vi "test Loopback BC to RT with Start and Stop.vi"(8 "error in":errorcluster, 11 "TestCase in":refnum<class "Loopback.lvclass">) -> (0 "error out":errorcluster, 3 "TestCase out":refnum<class "Loopback.lvclass">)   [LabVIEW 2020, in "Loopback.lvclass"]
uses:
  Loopback.lvclass
  C:/Git/niveristand-custom-device-testing-tools/VeriStandTestCase/VeriStandTestCase.lvclass
  <vilib>/numeric/Random Number (Range) U64.vi
  485b7c2b-8320-4722-9ec7-d01f27c65546.vi
  b08989c6-5f8b-4abd-9880-ddf65696a96d.vi
  632f36f1-4b6f-4095-917c-563c19b80c3a.vi
  c8f491d9-e213-4f8e-8b18-a73afe23b1be.vi
  0f9dda61-2c21-4955-8588-a8fc95227647.vi
  33c3b3d1-f053-43c7-bbe8-20c4ad88f1fe.vi
  757b3fb2-d48b-4fbb-8961-a38cd8e327a9.vi
  ff2cfcab-6673-4a18-a151-e28207f633c9.vi
  9a38d044-f7fa-4f05-ac83-bb7c785194b9.vi
  <vilib>/numeric/sub_Random U32.vi
  <vilib>/NI VeriStand/Execution/Workspace/NI VeriStand - Set Multiple Channel Values.vi
  <vilib>/NI VeriStand/Execution/Workspace/NI VeriStand - Get Multiple Channel Values.vi
  <vilib>/NI VeriStand/Execution/Workspace/NI VeriStand - Set Single Channel Value.vi
  <vilib>/addons/_JKI Toolkits/VI Tester/TestCase.llb/TestCase.lvclass
  <vilib>/NI VeriStand/Execution/Workspace/NI_VS Workspace ExecutionAPI.lvlib
  C:/Program Files (x86)/National Instruments/LabVIEW 2020/vi.lib/addons/_JKI Toolkits/VI Tester/TestCase.llb/TestCase.lvclass
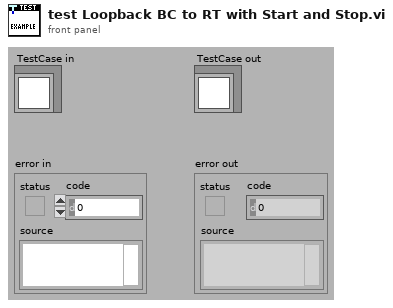
[diagram p1: front panel]
types:
  T1 = typedef "NI_VS Workspace ExecutionAPI.lvlib/WorkspaceAPI.ctl" = refnum<k24>
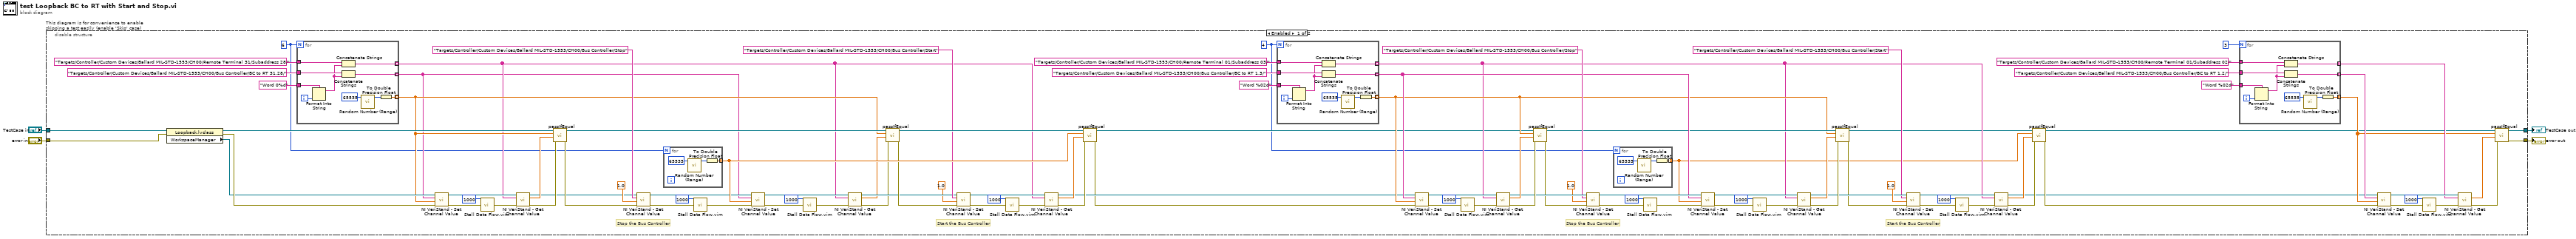
[diagram p0: block diagram]
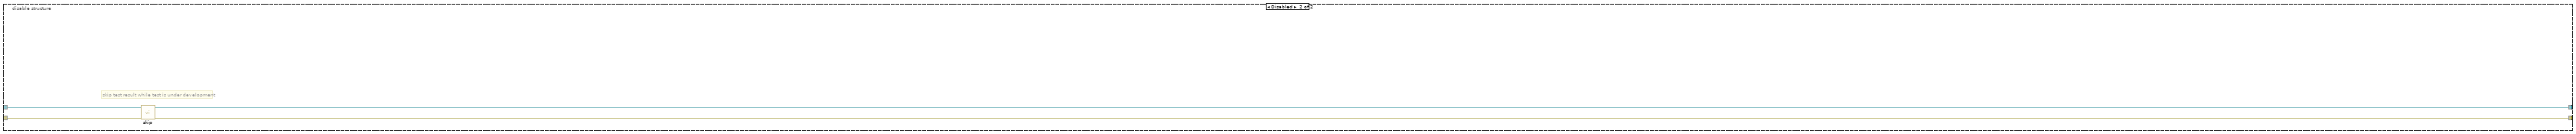
[diagram p2: hidden frame]
diagram:
  n1 = disable-structure "This diagram is for convenience to enable skipping a test easily (enable 'Skip' case)" shown="Enabled" {
    disable-tunnel: "TestCase in" -> [w101 w150]
    disable-tunnel: [w74 w148] -> w1
    disable-tunnel: [w73 w149] -> w3
    disable-tunnel: "error in" -> [w98 w147]
    frame Enabled {
      w5 = 4
      w6 = 6
      # "Start the Bus Controller"
      # "Stop the Bus Controller"
      # "Start the Bus Controller"
      # "Stop the Bus Controller"
      n2 = property class="Loopback.lvclass"(reference=w101, error in=w98) -> (reference out=w110:refnum<class "Loopback.lvclass">, error out=w105:errorcluster, "WorkspaceManager"=w103:T1)
      n3 = for {
        N: w6 -> [_]
        tunnel: "Targets/Controller/Custom Devices/Ballard MIL-STD-1553/CH00/Bus Controller/BC to RT 31.28/" ("Channel") -> [w145]
        tunnel: [w146] -> w8 mode=indexing
        tunnel: "Targets/Controller/Custom Devices/Ballard MIL-STD-1553/CH00/Remote Terminal 31/Subaddress 28/" ("Channel") -> [w144]
        tunnel: [w143] -> w9 mode=indexing
        tunnel: "Word 0%d" -> [w141]
        tunnel: [w137] -> w10 mode=indexing
        i -> [w142]
        n4 = Format Into String(format string=w141, w142) -> (resulting string=w140:string)  [unwired: 2 in, 1 out]
        n5 = Concatenate Strings(w144, w140) -> (w143:string)
        n6 = Concatenate Strings(w145, w140) -> (w146:string)
        n7 = call-poly <vilib>:"Random Number (Range).vi"("upper bound (100)"=u64 65535) -> ("number"=w139:u64)  [unwired: 10 in]
        n8 = To Double Precision Float(number=w139) -> (double precision float=w137:dbl)
      }
      n9 = call-poly <vilib>:"NI VeriStand - Set Channel Value.vi"("error in (no error)"=w105, "Values"=w10, "Channels"=w8, "WorkspaceManager in"=w103) -> ("error out"=w107:errorcluster, "WorkspaceManager out"=w109:T1)  [unwired: 6 in]
      n10 = call "Stall Data Flow.vim"("value in"=w107, "milliseconds to wait"=u32 1000) -> ("value out"=w108:errorcluster)  [unwired: 1 out]
      n11 = call-poly <vilib>:"NI VeriStand - Get Channel Value.vi"("error in (no error)"=w108, "Channels"=w9, "WorkspaceManager in"=w109) -> ("error out"=w104:errorcluster, "Values"=w102:dbl[], "WorkspaceManager out"=w12:T1)  [unwired: 6 in]
      n12 = call-dynamic "passIfEqual.vi"("error in (no error)"=w104, "y"=w102, "x"=w10, "TestCase in"=w110) -> ("error out"=w13:errorcluster, "TestCase out"=w11:refnum<class "Loopback.lvclass">)  [unwired: 6 in]
      n13 = call-poly <vilib>:"NI VeriStand - Set Channel Value.vi"("error in (no error)"=w13, "Value"=1.0, "Channel"="Targets/Controller/Custom Devices/Ballard MIL-STD-1553/CH00/Bus Controller/Stop", "WorkspaceManager in"=w12) -> ("error out"=w38:errorcluster, "WorkspaceManager out"=w18:T1)  [unwired: 6 in]
      n14 = for {
        N: w6 -> [_]
        tunnel: [w134] -> w32 mode=indexing
        n15 = call-poly <vilib>:"Random Number (Range).vi"("upper bound (100)"=u64 65535) -> ("number"=w135:u64)  [unwired: 10 in]
        n16 = To Double Precision Float(number=w135) -> (double precision float=w134:dbl)
      }
      n17 = call "Stall Data Flow.vim"("value in"=w38, "milliseconds to wait"=u32 1000) -> ("value out"=w39:errorcluster)  [unwired: 1 out]
      n18 = call-poly <vilib>:"NI VeriStand - Set Channel Value.vi"("error in (no error)"=w39, "Values"=w32, "Channels"=w8, "WorkspaceManager in"=w18) -> ("error out"=w34:errorcluster, "WorkspaceManager out"=w19:T1)  [unwired: 6 in]
      n19 = call "Stall Data Flow.vim"("value in"=w34, "milliseconds to wait"=u32 1000) -> ("value out"=w35:errorcluster)  [unwired: 1 out]
      n20 = call-poly <vilib>:"NI VeriStand - Get Channel Value.vi"("error in (no error)"=w35, "Channels"=w9, "WorkspaceManager in"=w19) -> ("error out"=w20:errorcluster, "Values"=w21:dbl[], "WorkspaceManager out"=w23:T1)  [unwired: 6 in]
      n21 = call-dynamic "passIfEqual.vi"("error in (no error)"=w20, "y"=w21, "x"=w10, "TestCase in"=w11) -> ("error out"=w27:errorcluster, "TestCase out"=w36:refnum<class "Loopback.lvclass">)  [unwired: 6 in]
      n22 = call-poly <vilib>:"NI VeriStand - Set Channel Value.vi"("error in (no error)"=w27, "Value"=1.0, "Channel"="Targets/Controller/Custom Devices/Ballard MIL-STD-1553/CH00/Bus Controller/Start", "WorkspaceManager in"=w23) -> ("error out"=w26:errorcluster, "WorkspaceManager out"=w31:T1)  [unwired: 6 in]
      n23 = call "Stall Data Flow.vim"("value in"=w26, "milliseconds to wait"=u32 1000) -> ("value out"=w30:errorcluster)  [unwired: 1 out]
      n24 = call-poly <vilib>:"NI VeriStand - Get Channel Value.vi"("error in (no error)"=w30, "Channels"=w9, "WorkspaceManager in"=w31) -> ("error out"=w29:errorcluster, "Values"=w28:dbl[], "WorkspaceManager out"=w14:T1)  [unwired: 6 in]
      n25 = call-dynamic "passIfEqual.vi"("error in (no error)"=w29, "y"=w28, "x"=w32, "TestCase in"=w36) -> ("error out"=w7:errorcluster, "TestCase out"=w15:refnum<class "Loopback.lvclass">)  [unwired: 6 in]
      n26 = for {
        N: w5 -> [_]
        tunnel: "Targets/Controller/Custom Devices/Ballard MIL-STD-1553/CH00/Bus Controller/BC to RT 1.3/" ("Channel") -> [w132]
        tunnel: [w133] -> w67 mode=indexing
        tunnel: "Targets/Controller/Custom Devices/Ballard MIL-STD-1553/CH00/Remote Terminal 01/Subaddress 03/" ("Channel") -> [w131]
        tunnel: [w130] -> w51 mode=indexing
        tunnel: "Word %02d" -> [w128]
        tunnel: [w124] -> w62 mode=indexing
        i -> [w129]
        n27 = Format Into String(format string=w128, w129) -> (resulting string=w127:string)  [unwired: 2 in, 1 out]
        n28 = Concatenate Strings(w131, w127) -> (w130:string)
        n29 = Concatenate Strings(w132, w127) -> (w133:string)
        n30 = call-poly <vilib>:"Random Number (Range).vi"("upper bound (100)"=u64 65535) -> ("number"=w126:u64)  [unwired: 10 in]
        n31 = To Double Precision Float(number=w126) -> (double precision float=w124:dbl)
      }
      n32 = call-poly <vilib>:"NI VeriStand - Set Channel Value.vi"("error in (no error)"=w7, "Values"=w62, "Channels"=w67, "WorkspaceManager in"=w14) -> ("error out"=w90:errorcluster, "WorkspaceManager out"=w88:T1)  [unwired: 6 in]
      n33 = call "Stall Data Flow.vim"("value in"=w90, "milliseconds to wait"=u32 1000) -> ("value out"=w89:errorcluster)  [unwired: 1 out]
      n34 = call-poly <vilib>:"NI VeriStand - Get Channel Value.vi"("error in (no error)"=w89, "Channels"=w51, "WorkspaceManager in"=w88) -> ("error out"=w92:errorcluster, "Values"=w93:dbl[], "WorkspaceManager out"=w72:T1)  [unwired: 6 in]
      n35 = call-dynamic "passIfEqual.vi"("error in (no error)"=w92, "y"=w93, "x"=w62, "TestCase in"=w15) -> ("error out"=w71:errorcluster, "TestCase out"=w65:refnum<class "Loopback.lvclass">)  [unwired: 6 in]
      n36 = call-poly <vilib>:"NI VeriStand - Set Channel Value.vi"("error in (no error)"=w71, "Value"=1.0, "Channel"="Targets/Controller/Custom Devices/Ballard MIL-STD-1553/CH00/Bus Controller/Stop", "WorkspaceManager in"=w72) -> ("error out"=w41:errorcluster, "WorkspaceManager out"=w68:T1)  [unwired: 6 in]
      n37 = for {
        N: w5 -> [_]
        tunnel: [w121] -> w50 mode=indexing
        n38 = call-poly <vilib>:"Random Number (Range).vi"("upper bound (100)"=u64 65535) -> ("number"=w122:u64)  [unwired: 10 in]
        n39 = To Double Precision Float(number=w122) -> (double precision float=w121:dbl)
      }
      n40 = call "Stall Data Flow.vim"("value in"=w41, "milliseconds to wait"=u32 1000) -> ("value out"=w40:errorcluster)  [unwired: 1 out]
      n41 = call-poly <vilib>:"NI VeriStand - Set Channel Value.vi"("error in (no error)"=w40, "Values"=w50, "Channels"=w67, "WorkspaceManager in"=w68) -> ("error out"=w48:errorcluster, "WorkspaceManager out"=w66:T1)  [unwired: 6 in]
      n42 = call "Stall Data Flow.vim"("value in"=w48, "milliseconds to wait"=u32 1000) -> ("value out"=w47:errorcluster)  [unwired: 1 out]
      n43 = call-poly <vilib>:"NI VeriStand - Get Channel Value.vi"("error in (no error)"=w47, "Channels"=w51, "WorkspaceManager in"=w66) -> ("error out"=w64:errorcluster, "Values"=w63:dbl[], "WorkspaceManager out"=w60:T1)  [unwired: 6 in]
      n44 = call-dynamic "passIfEqual.vi"("error in (no error)"=w64, "y"=w63, "x"=w62, "TestCase in"=w65) -> ("error out"=w56:errorcluster, "TestCase out"=w46:refnum<class "Loopback.lvclass">)  [unwired: 6 in]
      n45 = call-poly <vilib>:"NI VeriStand - Set Channel Value.vi"("error in (no error)"=w56, "Value"=1.0, "Channel"="Targets/Controller/Custom Devices/Ballard MIL-STD-1553/CH00/Bus Controller/Start", "WorkspaceManager in"=w60) -> ("error out"=w57:errorcluster, "WorkspaceManager out"=w52:T1)  [unwired: 6 in]
      n46 = call "Stall Data Flow.vim"("value in"=w57, "milliseconds to wait"=u32 1000) -> ("value out"=w53:errorcluster)  [unwired: 1 out]
      n47 = call-poly <vilib>:"NI VeriStand - Get Channel Value.vi"("error in (no error)"=w53, "Channels"=w51, "WorkspaceManager in"=w52) -> ("error out"=w54:errorcluster, "Values"=w55:dbl[], "WorkspaceManager out"=w43:T1)  [unwired: 6 in]
      n48 = call-dynamic "passIfEqual.vi"("error in (no error)"=w54, "y"=w55, "x"=w50, "TestCase in"=w46) -> ("error out"=w44:errorcluster, "TestCase out"=w45:refnum<class "Loopback.lvclass">)  [unwired: 6 in]
      n49 = for {
        N: 3 -> [_]
        tunnel: "Targets/Controller/Custom Devices/Ballard MIL-STD-1553/CH00/Bus Controller/BC to RT 1.2/" ("Channel") -> [w119]
        tunnel: [w120] -> w80 mode=indexing
        tunnel: "Targets/Controller/Custom Devices/Ballard MIL-STD-1553/CH00/Remote Terminal 01/Subaddress 02/" ("Channel") -> [w118]
        tunnel: [w117] -> w78 mode=indexing
        tunnel: "Word %02d" -> [w115]
        tunnel: [w111] -> w75 mode=indexing
        i -> [w116]
        n50 = Format Into String(format string=w115, w116) -> (resulting string=w114:string)  [unwired: 2 in, 1 out]
        n51 = Concatenate Strings(w118, w114) -> (w117:string)
        n52 = Concatenate Strings(w119, w114) -> (w120:string)
        n53 = call-poly <vilib>:"Random Number (Range).vi"("upper bound (100)"=u64 65535) -> ("number"=w113:u64)  [unwired: 10 in]
        n54 = To Double Precision Float(number=w113) -> (double precision float=w111:dbl)
      }
      n55 = call-poly <vilib>:"NI VeriStand - Set Channel Value.vi"("error in (no error)"=w44, "Values"=w75, "Channels"=w80, "WorkspaceManager in"=w43) -> ("error out"=w85:errorcluster, "WorkspaceManager out"=w87:T1)  [unwired: 6 in]
      n56 = call "Stall Data Flow.vim"("value in"=w85, "milliseconds to wait"=u32 1000) -> ("value out"=w86:errorcluster)  [unwired: 1 out]
      n57 = call-poly <vilib>:"NI VeriStand - Get Channel Value.vi"("error in (no error)"=w86, "Channels"=w78, "WorkspaceManager in"=w87) -> ("error out"=w83:errorcluster, "Values"=w82:dbl[])  [unwired: 6 in, 1 out]
      n58 = call-dynamic "passIfEqual.vi"("error in (no error)"=w83, "y"=w82, "x"=w75, "TestCase in"=w45) -> ("error out"=w73:errorcluster, "TestCase out"=w74:refnum<class "Loopback.lvclass">)  [unwired: 6 in]
    }
    frame Disabled {
      # "skip test result while test is under development"
      n59 = call <vilib>:"skip.vi"("error in (no error)"=w147, "TestCase in"=w150) -> ("error out"=w149:errorcluster, "TestCase out"=w148:refnum<class "Loopback.lvclass">)  [unwired: 8 in]
    }
  }
  "error out" <- w3
  "TestCase out" <- w1
